vi "Reset_gyro2.vi"(5 "Características Iniciais":T3={"Colors and Directions"=[enum."Zero", enum."Zero", enum."Zero", enum."Zero", enum."Zero", enum."Zero"], "Direction"=enum."Right", "CS"=enum."Street", "Old Color"=enum."White"}, 6 "NXT/EV3":T2, 7 "Parâmetros Iniciais":T5={"Gyro Port"=0, "Sensor - Left"=3, "Sensor - Right"=2, "     Color \nSensor Port"=1, "Kp Front"=0.5, "Motor speed"=-15, "Distance to street"=0.0, "Motor speed turns"=16, "Kp Curvas"=0.3} {"Kp Front" format="%.3f"; "Color \nSensor Port" items=["Port 1", "Port 2", "Port 3", "Port 4"]; "Sensor - Right" items=["Port 1", "Port 2", "Port 3", "Port 4"]; "Sensor - Left" items=["Port 1", "Port 2", "Port 3", "Port 4"]; "Gyro Port" items=["Port 1", "Port 2", "Port 3", "Port 4"]}, 9 "CS":T1(ring)=enum."Delivery", 10 "First Angle IN":sgl) -> (2 "First Angle OUT":sgl)   [LabVIEW 2016]
uses:
  parametros.ctl
  <vilib>/NXT/Block Support/NXT_InputPort.ctl
  caracteristicas.ctl
  <vilib>/NXT/Subs/ColorSensorColors.ctl
  <vilib>/NXT/Subs/LVHSConnector.ctl
  <vilib>/NXT/LegoClasses/BrickReference/BrickReference.lvclass
  <vilib>/NXT/Dual Mode Library/Sensors/EV3_Gyro_Angle.vi
  <vilib>/NXT/NXTIO Xnodes/AddressXNode/NXTIOAddress.xnode
panel:
  # "black"
  # "blue"
  # "green"
  # "yellow"
  # "red"
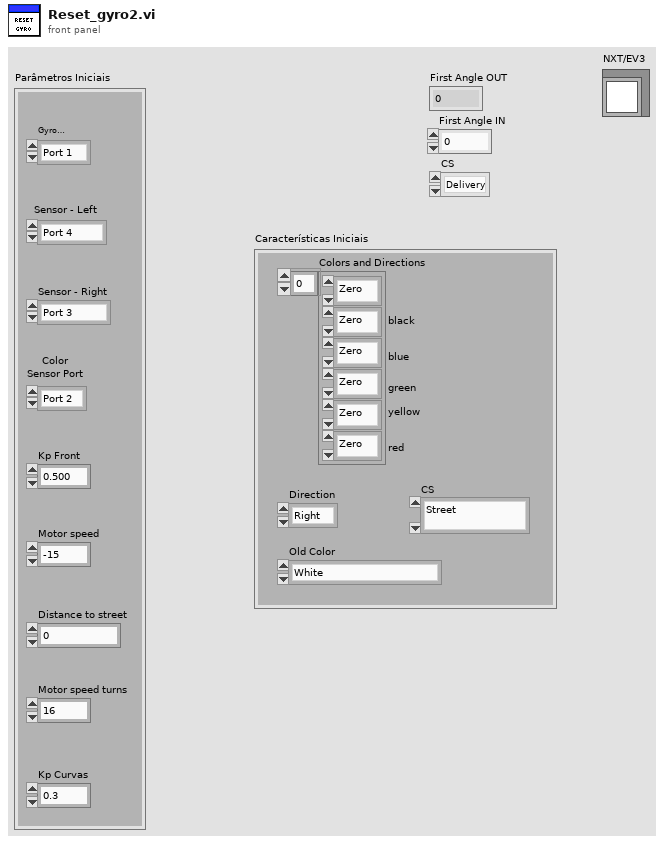
[diagram p1: front panel]
types:
  T1 = enum16{"Street", "Intersection", "End", "Stop", "Square", "Delivery"}
  T2 = typedef "LVHSConnector.ctl" = refnum<class "BrickReference.lvclass">
  T3 = typedef "caracteristicas.ctl" = cluster{"Colors and Directions":enum16{"Zero", "Right", "Front", "Left"}[], "Direction":enum16{"Zero", "Right", "Front", "Left"}, "CS":enum16{"Street", "Intersection", "End", "Stop", "Square", "Delivery", "Empty"}, "Old Color":T4}
  T4 = typedef "ColorSensorColors.ctl" = enum16{"No Color", "Black", "Blue", "Green", "Yellow", "Red", "White", "Brown"}
  T5 = typedef "parametros.ctl" = cluster{"Gyro Port":T6, "Sensor - Left":T6, "Sensor - Right":T6, "     Color \nSensor Port":T6, "Kp Front":dbl, "Motor speed":i32, "Distance to street":dbl, "Motor speed turns":i32, "Kp Curvas":dbl}
  T6 = typedef "NXT_InputPort.ctl" = u32
  T7 = enum16{"Street", "Intersection", "End", "Stop", "Square", "Delivery", "Empty"}
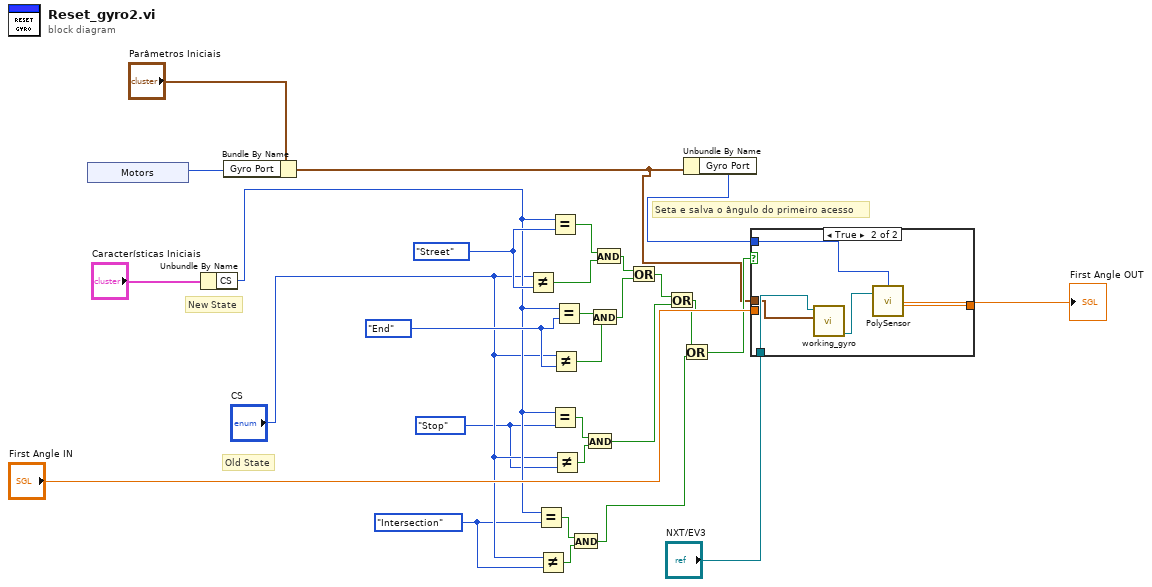
[diagram p0: block diagram]
diagram:
  w10 = T1."Intersection" ("CS")
  w9 = T1."Stop" ("CS")
  w26 = T1."End" ("CS")
  w29 = T1."Street" ("CS")
  # "New State"
  # "Old State"
  # "Seta e salva o ângulo do primeiro acesso"
  n1 = xnode "Motors"() -> ("Sensor"=w22:T6)
  n2 = Unbundle By Name("Características Iniciais") -> ("CS"=w12:T7)
  n3 = Bundle By Name(cluster="Parâmetros Iniciais", "Gyro Port"=w22) -> (w1:T5)
  n4 = Not Equal?(x="CS", y=w29) -> (x != y?=w27:bool)
  n5 = Equal?(x=w12, y=w10) -> (x = y?=w14:bool)
  n6 = Not Equal?(x="CS", y=w10) -> (x != y?=w13:bool)
  n7 = Equal?(x=w12, y=w29) -> (x = y?=w28:bool)
  n8 = Equal?(x=w12, y=w9) -> (x = y?=w16:bool)
  n9 = Not Equal?(x="CS", y=w26) -> (x != y?=w24:bool)
  n10 = Not Equal?(x="CS", y=w9) -> (x != y?=w15:bool)
  n11 = Equal?(x=w12, y=w26) -> (x = y?=w25:bool)
  n12 = And(x=w14, y=w13) -> (x .and. y?=w2:bool)
  n13 = And(x=w16, y=w15) -> (x .and. y?=w3:bool)
  n14 = And(x=w25, y=w24) -> (x .and. y?=w7:bool)
  n15 = And(x=w28, y=w27) -> (x .and. y?=w8:bool)
  n16 = Or(x=w8, y=w7) -> (x .or. y?=w6:bool)
  n17 = Or(x=w6, y=w3) -> (x .or. y?=w5:bool)
  n18 = Or(x=w5, y=w2) -> (x .or. y?=w4:bool)
  n19 = Unbundle By Name(w1) -> ("Gyro Port"=w21:T6)
  n20 = case shown="True" w4 {
    tunnel: "NXT/EV3" -> [_ w33]
    tunnel: [w30 w35] -> w19
    tunnel: "First Angle IN" -> [w30 _]
    tunnel: w21 -> [_ w34]
    tunnel: w1 -> [_ w31]
    frame False {
    }
    frame True {
      n21 = call "working_gyro.vi"("Parâmetros Iniciais"=w31, "NXT/EV3"=w33) -> ("NXT/EV3 2"=w32:T2)  [unwired: 9 in]
      n22 = call-poly <vilib>:"PolySensor.vi"("NXT/EV3"=w32, "Port (Port 1)"=w34) -> ("Degrees"=w35:sgl)  [unwired: 1 in, 1 out]
    }
  }
  "First Angle OUT" <- w19
